vi "Check if within limits.vi"(8 "error in (no error)":errorcluster, 10 "Target position array":dbl[](array[numeric]), 11 "ConfocalStage in":refnum<class "ConfocalStage.lvclass">) -> (0 "error out":errorcluster, 2 "in range?":bool, 3 "ConfocalStage out":refnum<class "ConfocalStage.lvclass">)   [LabVIEW 2012, in "ConfocalStage.lvclass"]
uses:
  ConfocalStage.lvclass
  ConfocalStage.lvclass/ConfocalStage.ctl
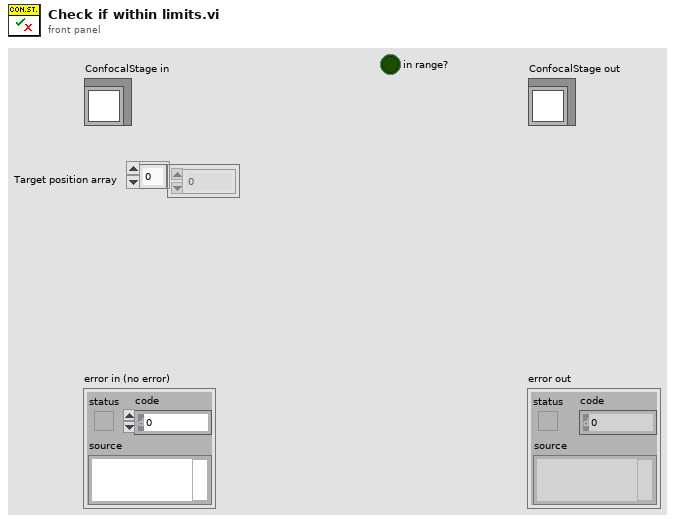
[diagram p1: front panel]
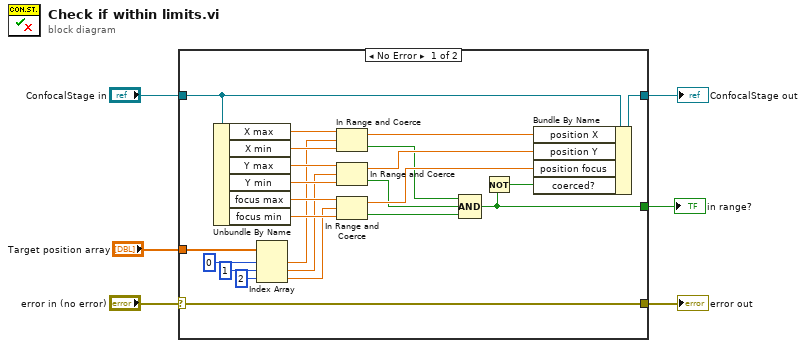
[diagram p0: block diagram]
diagram:
  n1 = case shown="No Error" "error in (no error)" {
    selector: "error in (no error)" -> [w30 w32]
    tunnel: [w30 w32] -> w5
    tunnel: [w22 w31] -> w3
    tunnel: "ConfocalStage in" -> [w23 w31]
    tunnel: [w8 _] -> w2
    tunnel: "Target position array" -> [w15 _]
    frame No Error {
      n2 = Unbundle By Name(w23) -> ("X max"=w29:dbl, "X min"=w28:dbl, "Y max"=w27:dbl, "Y min"=w26:dbl, "focus max"=w25:dbl, "focus min"=w24:dbl)
      n3 = Index Array(array=w15, index #1=0 ("index"), index #2=1 ("index"), index #3=2 ("index")) -> (element #1=w11:dbl, element #2=w10:dbl, element #3=w9:dbl)
      n4 = In Range and Coerce(upper limit=w29, x=w11, lower limit=w28) -> (coerced(x)=w21:dbl, In Range?=w18:bool)
      n5 = In Range and Coerce(upper limit=w27, x=w10, lower limit=w26) -> (coerced(x)=w20:dbl, In Range?=w17:bool)
      n6 = In Range and Coerce(upper limit=w25, x=w9, lower limit=w24) -> (coerced(x)=w19:dbl, In Range?=w16:bool)
      n7 = Compound Arithmetic op=AND(w18, w17, w16) -> (w8:bool)
      n8 = Not(x=w8) -> (.not. x?=w7:bool)
      n9 = Bundle By Name(cluster=w23, "position X"=w21, "position Y"=w20, "position focus"=w19, "coerced?"=w7) -> (w22:refnum<class "ConfocalStage.lvclass">)
    }
    frame Error {
    }
  }
  "error out" <- w5
  "ConfocalStage out" <- w3
  "in range?" <- w2
